vi "ClusterObtainRefs.vi"(6 "Add Cluster Name?":bool, 7 "caller name":string, 8 "error in (no error)":errorcluster, 11 "Clust Refnum":refnum<vi>) -> (0 "error out":errorcluster, 3 "Ref cluster":T1)   [LabVIEW 2025, in "UI_Library.lvlib" / "UI_Library.lvclass"]
uses:
  UI_Library.lvclass
  Controls/UI_RefCluster.ctl
  <vilib>/Utility/Data Type/Type Definitions/Data Type.ctl
  <vilib>/Utility/Data Type/NI_Data Type.lvlib
  UI_Library.lvlib
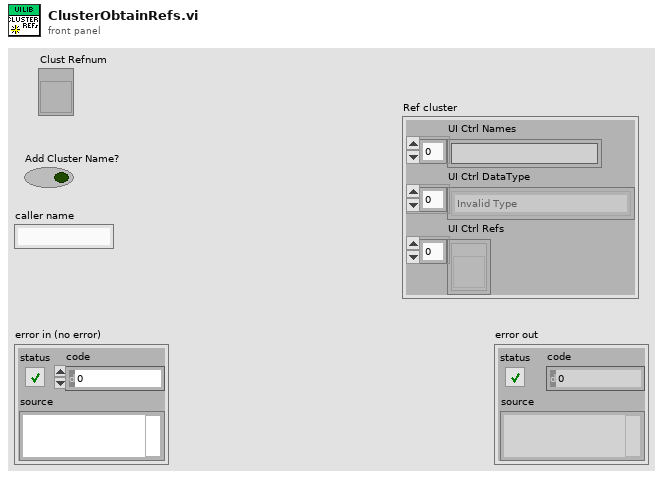
[diagram p1: front panel]
types:
  T1 = typedef "UI_Library.lvlib/UI_RefCluster.ctl" = cluster{"UI Ctrl Names":string[], "UI Ctrl DataType":T2[], "UI Ctrl Refs":refnum<vi>[]}
  T2 = typedef "NI_Data Type.lvlib/Data Type.ctl" = enum8{"Invalid Type", "Void", "I8", "I16", "I32", "I64", "U8", "U16", "U32", "U64", "Single Float", "Double Float", "Extended Float", "Single Complex", "Double Complex", "Extended Complex", "Enum U8", "Enum U16", "Enum U32", "Enum U64", "Single Float With Unit", "Double Float With Unit", "Extended Float With Unit", "Single Complex with Unit", "Double Complex with Unit", "Extended Complex with Unit", "Boolean", "String", "Path", "Picture", "Tag", "Array", "Cluster", "Variant", "LV Variant", "Waveform", "Timestamp", "Digital Waveform", "Digital Data", "ExpressData", "Refnum", "External Data", "VI", "Poly VI", "LabVIEW Class Instance", "Fixed Point", "Set Collection", "Map Collection"}
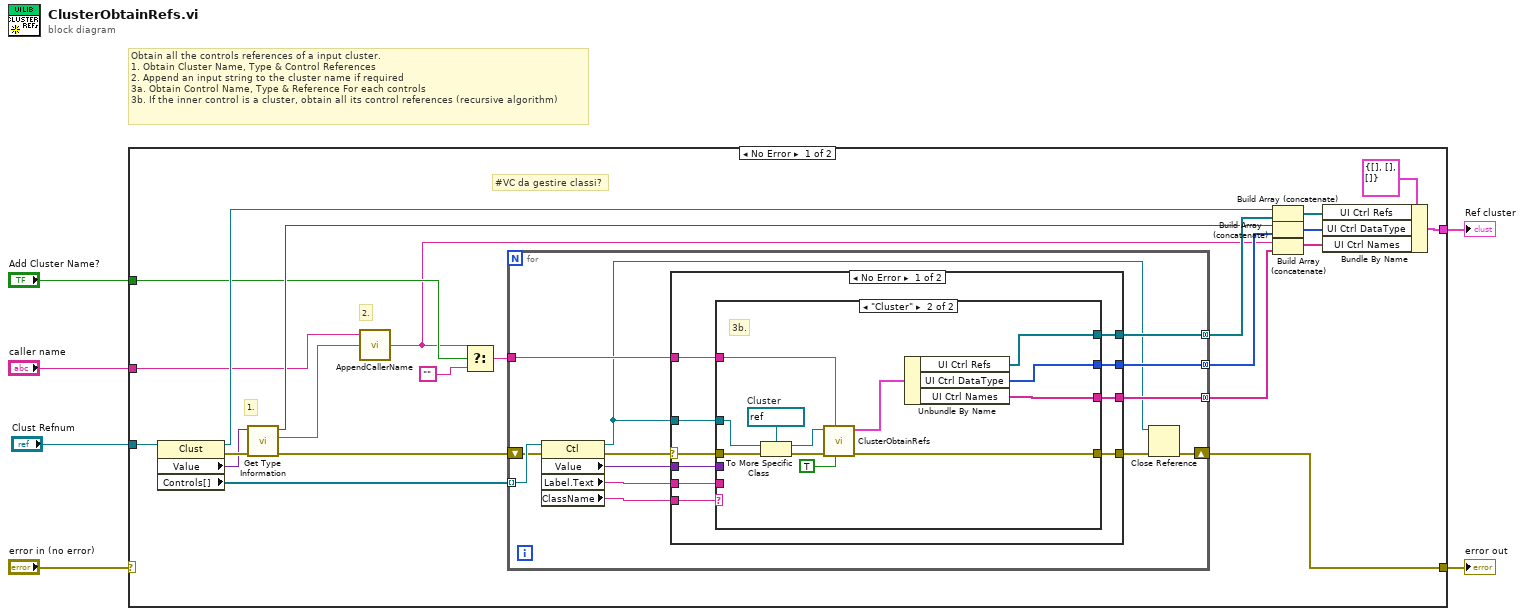
[diagram p0: block diagram]
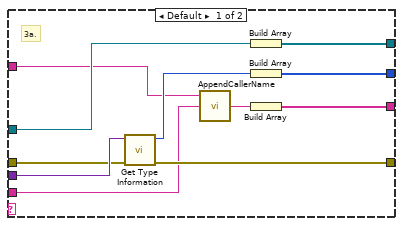
[diagram p2: hidden frame]
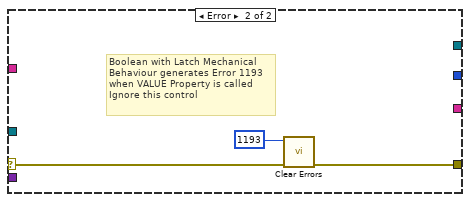
[diagram p3: hidden frame]
diagram:
  # "Obtain all the controls references of a input cluster.\n1. Obtain Cluster Name, Type & Control References\n2. Append an input string to the cluster name if required\n3a. Obtain Control Name, Type & Reference For each controls\n3b. If the inner control is a cluster, obtain all its control references (recursive algorithm)"
  n1 = case shown="No Error" "error in (no error)" {
    selector: "error in (no error)" -> [_ w78]
    tunnel: [w28 w78] -> w5
    tunnel: [w27 _] -> w4
    tunnel: "Clust Refnum" -> [w16 _]
    tunnel: "Add Cluster Name?" -> [w13 _]
    tunnel: "caller name" -> [w10 _]
    frame No Error {
      # "#VC da gestire classi?"
      # "2."
      # "1."
      n2 = property on="Property Node" class="Clust"(reference=w16) -> (reference out=w20:refnum<vi>, error out=w18:errorcluster, "Value"=w14:variant, "Controls[]"=w15:refnum<vi>[])  [unwired: 1 in]
      n3 = call <vilib>:"Get Type Information.vi"("error in (no error)"=w18, "variant"=w14) -> ("error out"=w17:errorcluster, "name"=w11:string, "type"=w19:T2)  [unwired: 5 in, 2 out]
      n4 = call "AppendCallerName.vi"("B"=w11, "A"=w10) -> ("A.B"=w8:string)  [unwired: 1 in]
      n5 = Select(t=w8, s=w13, f="") -> (s? t:f=w9:string)
      n6 = for {
        tunnel: w15 -> [w41] mode=indexing
        shift-right: [w31] -> w28
        shift-left: w17 -> [w40]
        tunnel: w9 -> [w39]
        tunnel: [w38] -> w21 mode=concatenating
        tunnel: [w37] -> w22 mode=concatenating
        tunnel: [w35] -> w12 mode=concatenating
        n7 = property on="Property Node" class="Ctl"(reference=w41, error in=w40) -> (reference out=w29:refnum<vi>, error out=w32:errorcluster, "Value"=w36:variant, "Label.Text"=w33:string, "ClassName"=w34:string)
        n8 = case shown="No Error" w32 {
          selector: w32 -> [w42 w76]
          tunnel: [w51 w77] -> w30
          tunnel: w29 -> [w50 _]
          tunnel: w39 -> [w49 _]
          tunnel: [w48 _] -> w38
          tunnel: [w47 _] -> w37
          tunnel: w36 -> [w46 _]
          tunnel: [w45 _] -> w35
          tunnel: w34 -> [w44 _]
          tunnel: w33 -> [w43 _]
          frame No Error {
            n9 = case shown="\"Cluster\"" w44 {
              tunnel: [w55 w74] -> w51
              tunnel: w42 -> [w56 w69]
              tunnel: w50 -> [w54 w70]
              tunnel: [w61 w67] -> w47
              tunnel: w49 -> [w53 w63]
              tunnel: [w60 w66] -> w48
              tunnel: w46 -> [w59 _]
              tunnel: [w57 w64] -> w45
              tunnel: w43 -> [w52 _]
              frame Default {
                # "3a."
                n10 = call <vilib>:"Get Type Information.vi"("error in (no error)"=w56, "variant"=w59) -> ("error out"=w55:errorcluster, "type"=w58:T2)  [unwired: 5 in, 3 out]
                n11 = call "AppendCallerName.vi"("B"=w52, "A"=w53) -> ("A.B"=w62:string)  [unwired: 1 in]
                n12 = Build Array(w54) -> (w60:refnum<vi>[])
                n13 = Build Array(w58) -> (w57:T2[])
                n14 = Build Array(w62) -> (w61:string[])
              }
              frame "Cluster" {
                w71 = refnum<vi> refnum  # Cluster
                # "3b."
                n15 = To More Specific Class(target class=w71, reference=w70, error in=w69) -> (specific class reference=w73:refnum<vi>, error out=w72:errorcluster)
                n16 = call "ClusterObtainRefs.vi"("Add Cluster Name?"=TRUE, "caller name"=w63, "error in (no error)"=w72, "Clust Refnum"=w73) -> ("error out"=w74:errorcluster, "Ref cluster"=w68:T1)  [unwired: 6 in]
                n17 = Unbundle By Name(w68) -> ("UI Ctrl Refs"=w66:refnum<vi>[], "UI Ctrl DataType"=w64:T2[], "UI Ctrl Names"=w67:string[])
              }
            }
          }
          frame Error {
            # "Boolean with Latch Mechanical\nBehaviour generates Error 1193 \nwhen VALUE Property is called\nIgnore this control"
            n18 = call <vilib>:"Clear Errors.vi"("error in (no error)"=w76, "specific error code to clear (0: all)"=1193) -> ("error out"=w77:errorcluster)  [unwired: 4 in, 1 out]
          }
        }
        n19 = Close Reference(reference=w29, error in (no error)=w30) -> (error out=w31:errorcluster)
      }
      n20 = Build Array (concatenate)(w20, w21) -> (w25:refnum<vi>[])
      n21 = Build Array (concatenate)(w19, w12) -> (w24:T2[])
      n22 = Build Array (concatenate)(w8, w22) -> (w23:string[])
      n23 = Bundle By Name(cluster=T1 {"UI Ctrl Names"=[], "UI Ctrl DataType"=[], "UI Ctrl Refs"=[]} ("UI-to-RT Ref cluster"), "UI Ctrl Refs"=w25, "UI Ctrl DataType"=w24, "UI Ctrl Names"=w23) -> (w27:T1)
    }
    frame Error {
    }
  }
  "error out" <- w5
  "Ref cluster" <- w4
